vi "Camera Manager Do Initialize.vi"(8 "error in (no error)":errorcluster) -> (0 "error out":errorcluster, 2 "function return":bool, 3 "CameraCount":i32[](array[numeric]))   [LabVIEW 2017, in "PlayNitrideCameraComponet1010_4.lvlib"]
doc: "__declspec(dllexport) bool CameraManager_DoInitialize(int* CameraCount);"
uses:
  <userlib>/PlayNitrideCameraComponet1010_4/PlayNitrideCameraComponet1010_4.lvlib
  <userlib>/PlayNitrideCameraComponet1010_4/PlayNitrideCameraComponet.dll
panel:
  # "__declspec(dllexport)  void CameraManager_GetCameraParam(int cameraId, char* NodeName, char* Value);"
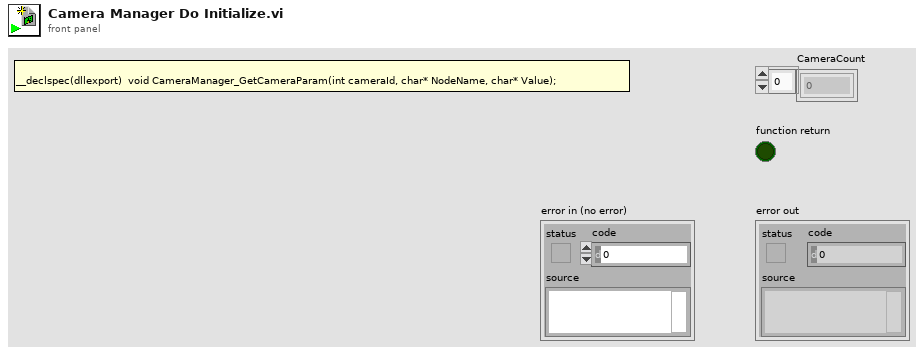
[diagram p1: front panel]
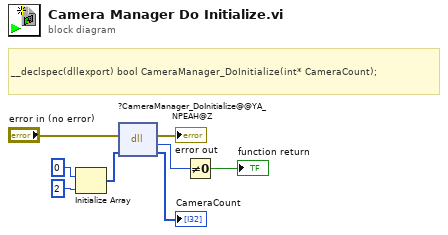
[diagram p0: block diagram]
diagram:
  # "__declspec(dllexport) bool CameraManager_DoInitialize(int* CameraCount);"
  n1 = Initialize Array(0 ("element"), 2 ("dimension size")) -> (w6:i32[])
  n2 = dll-call lib="C:/Program Files/National Instruments/LabVIEW 2017/user.lib/PlayNitrideCameraComponet1010_4/PlayNitrideCameraComponet.*" fn="?CameraManager_DoInitialize@@YA_NPEAH@Z"(error in="error in (no error)", "CameraCount"=w6) -> (error out=→"error out":errorcluster, "return type"=w7:u8, "CameraCount"=→"CameraCount":i32[])  [unwired: 2 in, 1 out]
  n3 = Not Equal To 0?(x=w7) -> (x != 0?=→"function return":bool)
